vi "Start Task-Points.vi"(8 "error in":errorcluster, 10 "Task Ident":string, 11 "Series Actor in":refnum<class "Series Actor.lvclass">) -> (0 "error out":errorcluster, 3 "Series Actor out":refnum<class "Series Actor.lvclass">)   [LabVIEW 2024, in "Series Actor.lvlib" / "Series Actor.lvclass"]
uses:
  Series Actor.lvclass
  Series Actor.lvclass/Series Actor.ctl
  <vilib>/ActorFramework/Message Enqueuer/Message Enqueuer.lvclass/Message Enqueuer.ctl
  <vilib>/ActorFramework/Message Enqueuer/Enqueue.vi
  Task/ITask Actor/ITask Actor Messages/Start Msg/Start Msg.lvclass
  <vilib>/Utility/LVClass/Get LV Class Name.vi
  <resource>/AFDebug/Generate Trace for Message.vi
  <vilib>/ActorFramework/Message Priority Queue/Priority Enqueue.vi
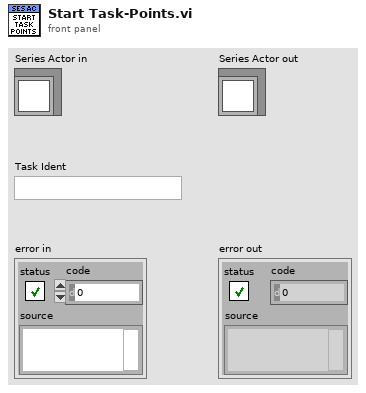
[diagram p1: front panel]
types:
  T1 = map{string, refnum<class "Message Enqueuer.lvclass">}
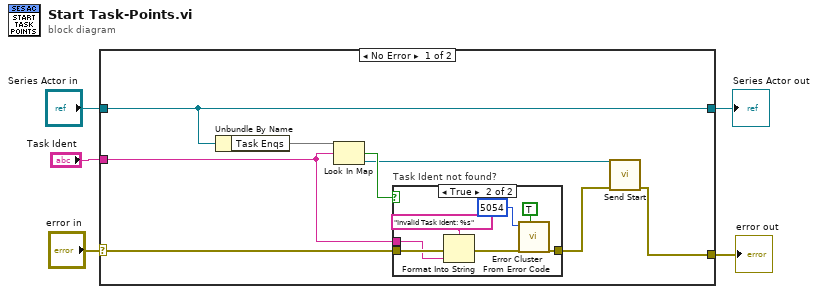
[diagram p0: block diagram]
diagram:
  n1 = case shown="No Error" "error in" {
    selector: "error in" -> [w8 w23]
    tunnel: [w7 w23] -> w4
    tunnel: [w9 w22] -> w2
    tunnel: "Series Actor in" -> [w9 w22]
    tunnel: "Task Ident" -> [w6 _]
    frame No Error {
      n2 = Unbundle By Name(w9) -> ("Task Enqs"=w13:T1)
      n3 = Look In Map(map=w13, key=w6) -> (key not found?=w12:bool, value=w10:refnum<class "Message Enqueuer.lvclass">)  [unwired: 1 in]
      n4 = case "Task Ident not found?" shown="True" w12 {
        tunnel: w8 -> [w14 w20]
        tunnel: [w14 w19] -> w11
        tunnel: w6 -> [_ w15]
        frame False {
        }
        frame True {
          n5 = Format Into String(format string="Invalid Task Ident: %s" ("error message (\"\")"), error in=w20, w15) -> (error out=w17:errorcluster)  [unwired: 1 in, 1 out]
          n6 = call <vilib>:"Error Cluster From Error Code.vi"("show call chain? (False)"=TRUE, "error in (no error)"=w17, "error code (0)"=5054) -> ("error out"=w19:errorcluster)  [unwired: 6 in]
        }
      }
      n7 = call "Send Start.vi"("error in (no error)"=w11, "Message Enqueuer"=w10) -> ("error out"=w7:errorcluster)  [unwired: 8 in, 1 out]
    }
    frame Error {
    }
  }
  "error out" <- w4
  "Series Actor out" <- w2
